vi "Dashboard Main.vi"() -> ()   [LabVIEW 2014]
uses:
  Program Files (x86)/National Instruments/LabVIEW 2014/examples/FRC/roboRIO/Vision/2015 Vision Example/Vision Support Code/Camera Types.ctl
  <vilib>/event_ctls.llb/eventvkey.ctl
  <vilib>/Rock Robotics/WPI/Dashboard/WPI_DashboardLogging Global.vi
  <vilib>/Rock Robotics/Network Tables/SD Write Number.vi
  <vilib>/Rock Robotics/Network Tables/SD Write Boolean.vi
  <vilib>/Utility/config.llb/Write Key (String).vi
  <vilib>/Utility/config.llb/Write Key (I32).vi
  <vilib>/Utility/config.llb/NI_LVConfig.lvlib
  <vilib>/vision/NI_Vision_Development_Module.lvlib
panel:
  out "Camera Image 6":T1(plugin-control)
  out "Image Message":string="Timeout in Camera Communications"
  in  "TCP":refnum<k5>
  in  "Rec Mode":enum32{"Stop", "Record", "Playback"}(radio)
  in  "Vision":u16(ring)=3 items=["Camera Off", "USB Camera SW", "USB Camera HW", "IP Camera"]
  out "Camera IP":string
  in  "Dashboard Tab":T2(tab)
  in  "Camera Settings":T3={"Frame Rate"=30, "Compression"=30, "Size"=1} {"Frame Rate" scale=1.0..30.0; "Size" items=["640x480", "320x240", "160x120"]}
  out "MotorChart R":cluster{"Numeric":dbl, "Numeric":dbl}(graph)
  out "MotorChart L":T4(graph)
  out "MotorSliders R":cluster{"MotorSlide1":dbl, "MotorSlide2":dbl} {"MotorSlide2" scale=-1.0..1.0 scale format="%#_2e"; "MotorSlide1" scale=-1.0..1.0 scale format="%#_2e"}
  out "MotorSliders L":T5 {"MotorSlide4 2" scale=0.0..14.0 scale format="%#_2e"; "MotorSlide2" scale=-1.0..1.0 scale format="%#_2e"; "MotorSlide1" scale=-1.0..1.0 scale format="%#_2e"}
  out "Gyro":dbl(knob) scale=0.0..360.0
  out "JS1 Z":dbl(slide) scale=-1.0..1.0 scale format="%#_2e"
  out "JS1 Graph":cluster{"X":dbl, "Y":dbl}[](graph)
  out "JS1 Buttons":T6
  out "JS2 Z":dbl(slide) scale=-1.0..1.0 scale format="%#_2e"
  out "JS2 Graph":cluster{"X":dbl, "Y":dbl}[](graph)
  out "JS2 Buttons":T6
  out "Mode":T7(ring)=enum."Auto Disabled"
  in  "DB Camera Config":bool
  out "fps":dbl format="%#.1g"
  out "Mbps":dbl format="%#.1g"
  out "Mbps 2":bool
  in  "Tiempo de Espera":dbl
  in  "Repetir":bool
  in  "Autonomo":dbl
  out "Found Totes":T8(array[cluster]) {"Normalized Rect"."Numeric 5" format="%#_2g"; "Normalized Rect"."Numeric 3" format="%#_2g"; "Normalized Rect"."Numeric 2" format="%#_2g"; "Normalized Rect"."Numeric" format="%#_2g"}
  out "Sorted Scores":T9(array[cluster]) {"Carpet" format="%#_3g"; "S" format="%#_3g"; "Trapezoid %" format="%#_3g"; "L" format="%#_3g"; "Area to CH" format="%#_3g"; "X" format="%#_3g"; "Y" format="%#_3g"}
  out "Detected Totes":T8(array[cluster]) {"Normalized Rect"."Numeric 5" format="%#_2g"; "Normalized Rect"."Numeric 3" format="%#_2g"; "Normalized Rect"."Numeric 2" format="%#_2g"; "Normalized Rect"."Numeric" format="%#_2g"}
  out "Sorted Scores Extracted":T9(array[cluster]) {"Carpet" format="%#_3g"; "S" format="%#_3g"; "Trapezoid %" format="%#_3g"; "L" format="%#_3g"; "Area to CH" format="%#_3g"; "X" format="%#_3g"; "Y" format="%#_3g"}
  out "Detected Totes Extracted":T8(array[cluster]) {"Normalized Rect"."Numeric 5" format="%#_2g"; "Normalized Rect"."Numeric 3" format="%#_2g"; "Normalized Rect"."Numeric 2" format="%#_2g"; "Normalized Rect"."Numeric" format="%#_2g"}
  out "ms to process":u32
  in  "Tote Color":T10={"Hue"={23.67058792990901, 53.0}, "Sat"={88.0, 255.0}, "Val"={60.0, 159.85714285714286}} {"Hue" scale=0.0..255.0 scale format="%#_3g"}
  in  "Carpet Color":T11(tab)
  in  "Red":T10={"Hue"={231.0, 14.0}, "Sat"={83.0, 255.0}, "Val"={52.5, 255.0}} {"Hue" scale=0.0..255.0 scale format="%#_3g"}
  in  "Blue":T10={"Hue"={119.0, 181.0}, "Sat"={33.0, 255.0}, "Val"={48.571428571428584, 255.0}} {"Hue" scale=0.0..255.0 scale format="%#_3g"}
  in  "Annotate":bool=TRUE
  in  "Show Carpet Mask":bool=TRUE
  in  "Limit Tests?":bool=TRUE
  out "Particles":i32
  in  "Score Threshold":dbl=75.0
  in  "Aspect Fudge Factor":dbl=1.0
  in  "Camera Type":T12=enum."MS HD3000 square"
  out "Particles 2":i32
  in  "DB/String 9":string
  in  "DB/String 8":string
  in  "DB/String 7":string
  in  "DB/String 6":string
  in  "DB/String 5":string
  in  "DB/String 4":string
  in  "DB/String 3":string
  in  "DB/String 2":string
  in  "DB/String 1":string
  in  "DB/String 0":string
  in  "DB/Slider 0":dbl(slide) scale=0.0..5.0
  in  "DB/Slider 1":dbl(slide) scale=0.0..5.0
  in  "DB/Slider 2":dbl(slide) scale=0.0..5.0
  in  "DB/Slider 3":dbl(slide) scale=0.0..5.0
  out "DB/LED 3":bool
  out "DB/LED 2":bool
  out "DB/LED 1":bool
  out "DB/LED 0":bool
  in  "DB/Button 3":bool
  in  "DB/Button 2":bool
  in  "DB/Button 1":bool
  in  "DB/Button 0":bool caption="New Name"
  in  "Test Slider":dbl(slide) scale=0.0..100.0 scale format="%#_3g"
  in  "On/Off":bool caption="Solenoid"
  in  "Test Name":u16(ring) items=["Select the test to run...", "Example Test", "-------------------------------", "List of tests is built in robot code.", "Replace with your own automated tests."]
  in  "Test Tree":string(tree)
  in  "Motor":cluster{"Value":dbl, "Enable":bool} {"Value" scale=-1.0..1.0 scale format="%#_3g"}
  out "Progress":T13 {"Test Progress" scale=0.0..100.0}
  in  "Rev/Fwd":cluster{"Forward":bool, "Reverse":bool}
  in  "Test Ring":u16(ring) items=["Monochrome", "Color"]
  in  "Listbox":i32(listbox)
  out "Tree":string(tree)
  in  "Tab Control":T14(tab)
  out "Original Image":T1(plugin-control)
  out "Masked":T1(plugin-control)
  out "Original Extracted":T1(plugin-control)
  out "Extracted Masked":T1(plugin-control)
  out "Boolean":bool
  # "Left"
  # "Front"
  # "Right"
  # "Battery"
  # "Density Profile"
  # "Aspect Ratio"
  # "Density Profile"
  # "Aspect Ratio"
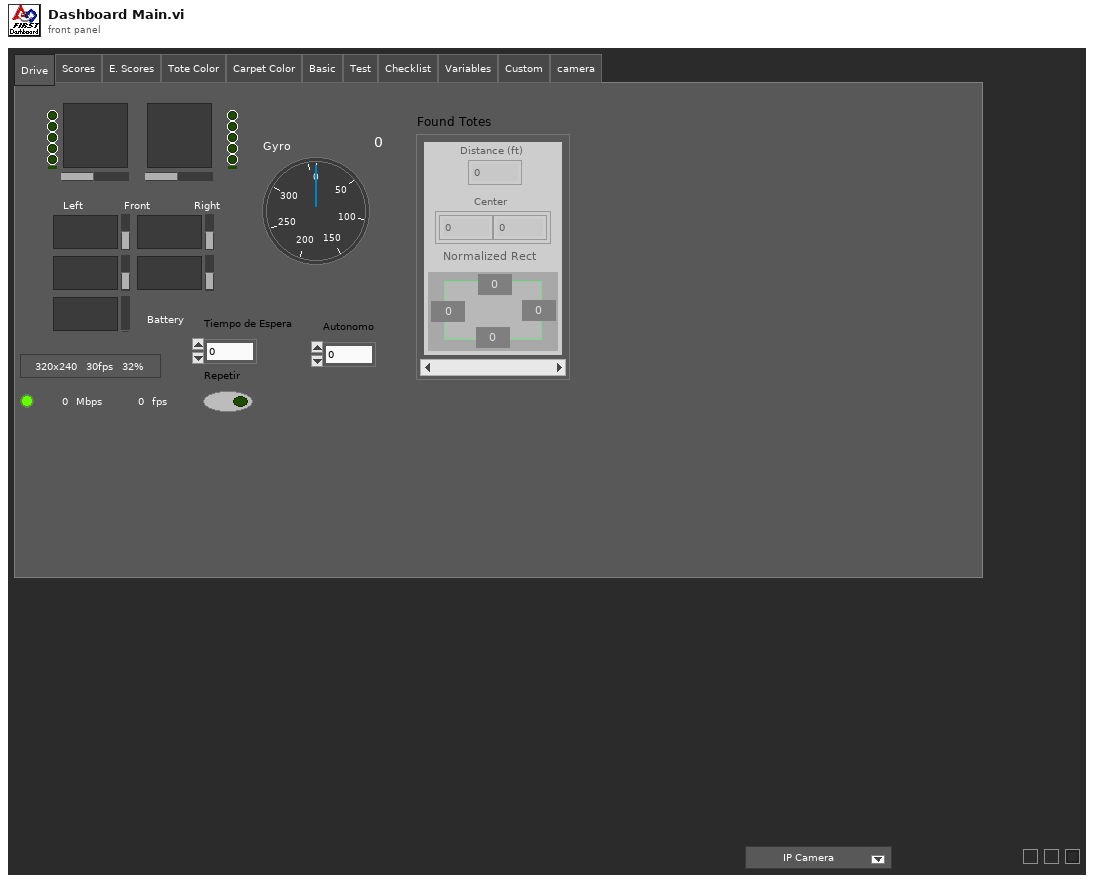
[diagram p1: front panel]
types:
  T1 = typedef "IMAQ Image.ctl" = refnum<image>
  T2 = enum32{"Drive", "Scores", "E. Scores", "Tote Color", "Carpet Color", "Basic", "Test", "Checklist", "Variables", "Custom", "camera"}
  T3 = cluster{"Frame Rate":i32, "Compression":i32, "Size":u16}
  T4 = cluster{"Numeric":dbl, "Numeric":dbl, "Battery V":dbl}
  T5 = cluster{"MotorSlide1":dbl, "MotorSlide2":dbl, "MotorSlide4 2":dbl}
  T6 = cluster{bool, bool, bool, bool, bool, bool, bool, bool, bool, bool, bool, bool}
  T7 = enum8{"Tele-Op Disabled", "Tele-Op Enabled", "Auto Disabled", "Auto Enabled", "Test Disabled", "Test Enabled", "Disconnected", "No Code", "E-Stop"}
  T8 = cluster{"Distance (ft)":dbl, "Center":cluster{dbl, dbl}, "Normalized Rect":cluster{"Numeric":dbl, "Numeric 2":dbl, "Numeric 3":dbl, "Numeric 5":dbl}}[]
  T9 = cluster{"Rectangle":cluster{"Numeric":dbl, "Numeric 2":dbl, "Numeric 3":dbl, "Numeric 5":dbl}, "Trapezoid %":dbl, "L":dbl, "S":dbl, "Area to CH":dbl, "X":dbl, "Y":dbl, "Carpet":dbl}[]
  T10 = cluster{"Hue":cluster{dbl, dbl}, "Sat":cluster{dbl, dbl}, "Val":cluster{dbl, dbl}}
  T11 = enum32{"Red Carpet Color", "Blue Carpet Color", "None"}
  T12 = typedef "Camera Types.ctl" = enum16{"206", "1011", "1013", "MS HD3000 square", "MS HD3000 640x480"}
  T13 = cluster{"Test Progress":u8, "Test Progress Text":string}
  T14 = enum32{"Original", "Masked", "Original Extracted", "Extracted Masked", "Rectangle"}
  T15 = typedef "Image Type" = u32
  T16 = typedef "Particle Parameters" = i32
  T17 = enum32{"Drive", "Basic", "Custom", "Test", "Checklist", "Variables"}
  T18 = cluster{"Camera Image 6":refnum<vi>, "Dashboard Tab":refnum<vi>, "Boolean":refnum<vi>, "Vision":refnum<vi>, "Rec Mode":refnum<vi>, "Test Slider":refnum<vi>, "On/Off ":refnum<vi>, "Test Ring":refnum<vi>, "Rev/Fwd":refnum<vi>, "Test Name":refnum<vi>, "Motor":refnum<vi>, "Progress":refnum<vi>, "CheckList":refnum<vi>, "Tree":refnum<vi>, "Test Tree":refnum<vi>}
  T19 = cluster{"Error Strings":string, "Disable Counts":cluster{u16, u16}, "Rail Faults":cluster{u16, u16, u16}, "Robot IP":string, "DB Mode":u8, "Event Info":cluster{"Name":string, "Type":u8, "Number":u16, "Replay":u8}, "Camera Addr":string}
  T20 = cluster{"Storage":cluster{"Disk Free":u64, "RAM Block":u32, "RAM free":u32}, "CPU Utilization":cluster{"CPU % ISR":sgl, "CPU % Time Crit":sgl, "CPU % Timed Str":sgl, "CPU % High":sgl, "CPU % Above":sgl, "CPU % Normal":sgl, "CPU % Low":sgl}, "CAN":cluster{"% Bus Utilization":sgl, "Bus Off Cnt":u32, "TX_FIFO Full Cnt":u32, "Receive Error Cnt":u8, "Transmit Error Cnt":u8}, "HID":cluster{"HID Outputs":u32, "Rumble Low":u16, "Rumble High":u16}[]}
  T21 = cluster{"Status bits":cluster{"Test Mode":bool, "Autonomous":bool, "Enabled":bool, "Code Start":bool, "Brownout":bool, "Reserved 2":bool, "Reserved 3":bool, "E-Stop":bool}, "Code Trace":cluster{"Disabled":bool, "TeleOp":bool, "Auto":bool, "Test":bool}, "Controller Type":enum16{"unknown", "cRIO", "roboRio"}, "Code?":enum16{"unknown", "noCode", "code"}, "Battery V":dbl}
  T22 = cluster{"Control Bits":cluster{"TestMode":bool, "Autonomous":bool, "Enabled":bool, "FMS Present":bool, bool, bool, bool, "E-Stop":bool}, "Team Station ":u8, "Countdown":sgl, "Joystick Values":cluster{"Axes":dbl[], "Buttons":bool[], "POVs":i16[]}[]}
  T23 = cluster{"Axes":dbl[], "Buttons":bool[], "POVs":i16[]}[]
  T24 = cluster{"Axes":dbl[], "Buttons":bool[], "POVs":i16[]}
  T25 = cluster{"Buttons[0]":bool, "Buttons[1]":bool, "Buttons[2]":bool, "Buttons[3]":bool, "Buttons[4]":bool, "Buttons[5]":bool, "Buttons[6]":bool, "Buttons[7]":bool, "Buttons[8]":bool, "Buttons[9]":bool, "Buttons[10]":bool, "Buttons[11]":bool}
  T26 = typedef "NI_LVConfig.lvlib/Config Data RefNum.ctl" = refnum<k1>
  T27 = cluster{"Operation":enum16{"Update", "Clear"}, "Color Box":u32}[]
  T28 = typedef "eventvkey.ctl" = enum16{"ASCII", "Enter", "Return", "Shift", "Ctrl", "Alt", "Cmd", "Opt", "Caps", "NumLock", "Clear", "Break", "Up", "Down", "Left", "Right", "Insert", "Delete", "Home", "End", "PageUp", "PageDown", "Escape", "Help", "Pause", "ScrollLock", "F1", "F2", "F3", "F4", "F5", "F6", "F7", "F8", "F9", "F10", "F11", "F12", "F13", "F14", "F15", "F16", "F17", "F18", "F19", "F20", "F21", "F22", "F23", "F24", "Play", "VolumeUp", "VolumeDown", "Mute", "Two Byte Char"}
  T29 = cluster{"Image Size":bool, "Image Type":bool, "Pixel Value":bool, "ROI Information":bool, "Zoom Factor":bool}
  T30 = enum8{"Enabled", "Disabled", "Disabled and Grayed Out"}
  T31 = cluster{"Operation":enum16{"Update", "Clear"}, "Color Box":u32}
  T32 = cluster{"Bounding box":cluster{"left":dbl, "top":dbl, "right":dbl, "bottom":dbl}, "Trapezoid":dbl, "Long Aspect":dbl, "Short Aspect":dbl, "Area to CH":dbl, "X Mask":dbl, "Y Mask":dbl, "Carpet":dbl}[]
  T33 = cluster{"Red":cluster{"Hue":cluster{dbl, dbl}, "Sat":cluster{dbl, dbl}, "Val":cluster{dbl, dbl}}, "Blue":cluster{"Hue":cluster{dbl, dbl}, "Sat":cluster{dbl, dbl}, "Val":cluster{dbl, dbl}}}
  T34 = cluster{cluster{"[0]":dbl, "[1]":dbl, "[2]":dbl, "[3]":dbl}, "Score":dbl, "Long Edge Score":dbl, "Short Edge Score":dbl, dbl, "X Score":dbl, "Y Score":dbl, "Carpet":dbl}[]
  T35 = cluster{"Found Totes[0]":cluster{"Distance (ft)":dbl, "Center":cluster{dbl, dbl}, "Normalized Rect":cluster{"Numeric":dbl, "Numeric 2":dbl, "Numeric 3":dbl, "Numeric 5":dbl}}, "Found Totes[1]":cluster{"Distance (ft)":dbl, "Center":cluster{dbl, dbl}, "Normalized Rect":cluster{"Numeric":dbl, "Numeric 2":dbl, "Numeric 3":dbl, "Numeric 5":dbl}}, "Found Totes[2]":cluster{"Distance (ft)":dbl, "Center":cluster{dbl, dbl}, "Normalized Rect":cluster{"Numeric":dbl, "Numeric 2":dbl, "Numeric 3":dbl, "Numeric 5":dbl}}, "Found Totes[3]":cluster{"Distance (ft)":dbl, "Center":cluster{dbl, dbl}, "Normalized Rect":cluster{"Numeric":dbl, "Numeric 2":dbl, "Numeric 3":dbl, "Numeric 5":dbl}}, "Found Totes[4]":cluster{"Distance (ft)":dbl, "Center":cluster{dbl, dbl}, "Normalized Rect":cluster{"Numeric":dbl, "Numeric 2":dbl, "Numeric 3":dbl, "Numeric 5":dbl}}, "Found Totes[5]":cluster{"Distance (ft)":dbl, "Center":cluster{dbl, dbl}, "Normalized Rect":cluster{"Numeric":dbl, "Numeric 2":dbl, "Numeric 3":dbl, "Numeric 5":dbl}}, "Found Totes[6]":cluster{"Distance (ft)":dbl, "Center":cluster{dbl, dbl}, "Normalized Rect":cluster{"Numeric":dbl, "Numeric 2":dbl, "Numeric 3":dbl, "Numeric 5":dbl}}, "Found Totes[7]":cluster{"Distance (ft)":dbl, "Center":cluster{dbl, dbl}, "Normalized Rect":cluster{"Numeric":dbl, "Numeric 2":dbl, "Numeric 3":dbl, "Numeric 5":dbl}}, "Found Totes[8]":cluster{"Distance (ft)":dbl, "Center":cluster{dbl, dbl}, "Normalized Rect":cluster{"Numeric":dbl, "Numeric 2":dbl, "Numeric 3":dbl, "Numeric 5":dbl}}}
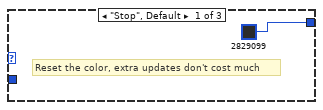
[diagram p3: hidden frame]
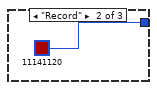
[diagram p4: hidden frame]
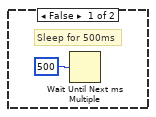
[diagram p6: hidden frame]
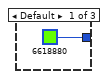
[diagram p7: hidden frame]
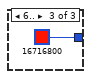
[diagram p8: hidden frame]
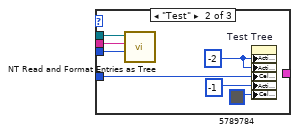
[diagram p10: hidden frame]
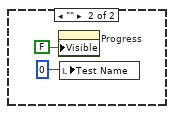
[diagram p11: hidden frame]
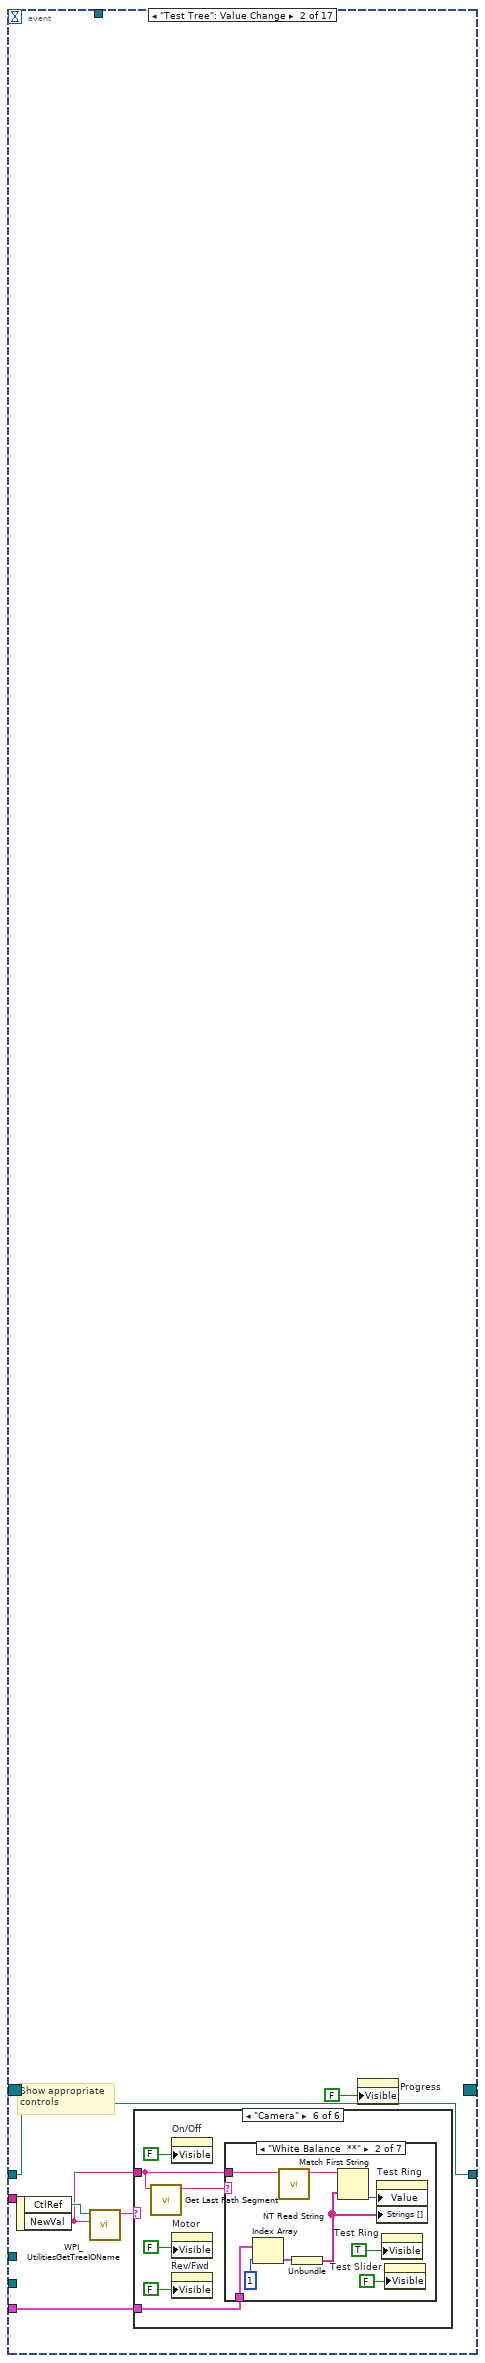
[diagram p12: hidden frame]
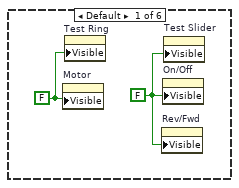
[diagram p13: hidden frame]
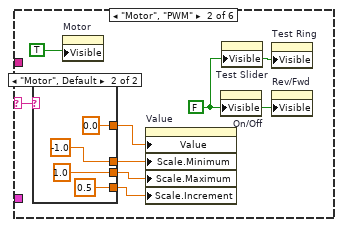
[diagram p14: hidden frame]
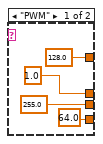
[diagram p15: hidden frame]
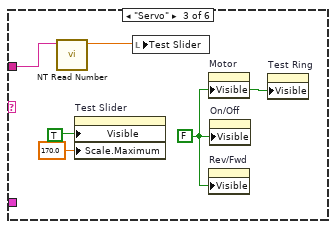
[diagram p16: hidden frame]
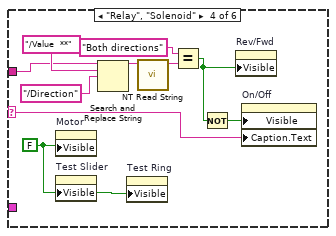
[diagram p17: hidden frame]
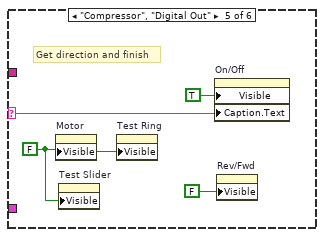
[diagram p18: hidden frame]
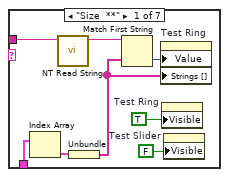
[diagram p19: hidden frame]
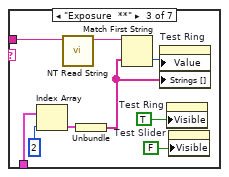
[diagram p20: hidden frame]
diagram:
  w5 = T15 0 items=["Grayscale (U8)", "Grayscale (I16)", "Grayscale (SGL)", "Complex (CSG)", "RGB (U32)", "HSL (U32)", "RGB (U64)"] ("Image Type")
  w7 = T15 4 items=["Grayscale (U8)", "Grayscale (I16)", "Grayscale (SGL)", "Complex (CSG)", "RGB (U32)", "HSL (U32)", "RGB (U64)", "Grayscale (U16)"] ("Image Type")
  w12 = T16[] [48, 35, 38, 4, 5, 6, 7, 0, 1, 2, 3] items=["Center of Mass X", "Center of Mass Y", "First Pixel X", "First Pixel Y", "Bounding Rect Left", "Bounding Rect Top", "Bounding Rect Right", "Bounding Rect Bottom", "Max Feret Diameter Start X", "Max Feret Diameter Start Y", "Max Feret Diameter End X", "Max Feret Diameter End Y", "Max Horiz. Segment Length Left", "Max Horiz. Segment Length Right", "Max Horiz. Segment Length Row", "-", "Bounding Rect Width", "Bounding Rect Height", "Bounding Rect Diagonal", "Perimeter", "Convex Hull Perimeter", "Holes' Perimeter", "Max Feret Diameter", "Equivalent Ellipse Major Axis", "Equivalent Ellipse Minor Axis", "Equivalent Ellipse Minor Axis (Feret)", "Equivalent Rect Long Side", "Equivalent Rect Short Side", "Equivalent Rect Diagonal", "Equivalent Rect Short Side (Feret)", "Average Horiz. Segment Length", "Average Vert. Segment Length", "Hydraulic Radius", "Waddel Disk Diameter", "-", "Area", "Holes' Area", "Particle & Holes' Area", "Convex Hull Area", "Image Area", "-", "Number of Holes", "Number of Horiz. Segments", "Number of Vert. Segments", "-", "Orientation", "Max Feret Diameter Orientation", "-", "% Area/Image Area", "% Area/(Particle & Holes' Area)", "Ratio of Equivalent Ellipse Axes", "Ratio of Equivalent Rect Sides", "-", "Elongation Factor", "Compactness Factor", "Heywood Circularity Factor", "Type Factor", "-", "Sum X", "Sum Y", "Sum XX", "Sum XY", "Sum YY", "Sum XXX", "Sum XXY", "Sum XYY", "Sum YYY", "-", "Moment of Inertia XX", "Moment of Inertia XY", "Moment of Inertia YY", "Moment of Inertia XXX", "Moment of Inertia XXY", "Moment of Inertia XYY", "Moment of Inertia YYY", "Norm. Moment of Inertia XX", "Norm. Moment of Inertia XY", "Norm. Moment of Inertia YY", "Norm. Moment of Inertia XXX", "Norm. Moment of Inertia XXY", "Norm. Moment of Inertia XYY", "Norm. Moment of Inertia YYY", "Hu Moment 1", "Hu Moment 2", "Hu Moment 3", "Hu Moment 4", "Hu Moment 5", "Hu Moment 6", "Hu Moment 7"]  # Requested Measurements
  w15 = T15 0 items=["Grayscale (U8)", "Grayscale (I16)", "Grayscale (SGL)", "Complex (CSG)", "RGB (U32)", "HSL (U32)", "RGB (U64)"] ("Image Type")
  w39 = 491  # min tab size
  w38 = 1.333  # min tab size
  w46 = enum32{"Stop", "Record", "Playback"}."Stop" ("Rec Mode")
  w22 = FALSE ("Visible")
  (unwired) "This VI has seven parallel loops for different tasks and a bit of initialization code that runs just once.\n\nTypical dashboard extensions only need to edit the panel. Adding new indicators or controls simply involves placing them on the panel in the Operations tab and naming them the same as the SmartDashboard variable on the robot\n\nIf the display needs to process the data before display, loop one is an example of doing that for the joysticks and motors.\n\nIf you want customize the video display or perform processing on it, loop two is where that takes place.\n\nOther loops should not need to be modified. They are pretty standard, and document the task they perform."  # Documentation
  w65 = T15 4 items=["Grayscale (U8)", "Grayscale (I16)", "Grayscale (SGL)", "Complex (CSG)", "RGB (U32)", "HSL (U32)", "RGB (U64)"] ("Image Type")
  # "Loop 7. Wait for DS connections"
  # "Basic debug and auto controls: Their data names are fixed, but\nthe displayed name, called a caption, can be changed directly or in\nrobot code such as shown in Begin."
  # "Controls for Test Mode, Camera Settings, etc."
  # "Additional UI Initialization"
  # "Loop 6. Animation for background of window during playback and record"
  # "Fires each time robot IP\nchanges, simulator does this"
  # "Fires each time window\ndocking changes."
  # "Collects all controls and indicators\nin the Basic and Custom tab.\nIf you need to bind additional controls,\nadd their references. You can extend the\nenum constant or use an integer."
  # "The remaining code below this line typically doesn't need to be modified."
  # "Loop 4. Process UI events related to test mode, checklist, and camera settings"
  # "Terminals of controls and indicators that are bound to the smart dashboard by name.\nYou can place the terminals anywhere you like and even read data from them.\nYou bind controls by adding the control reference to the array on the left. The subVI will\ndo this for the contents of a tab, and you can do it for individual items too, as shown with\nthe LED. To create get the reference, right-click and Create>>Reference."
  # "Loop 3. Wait until the robot response provides\n the Robot IP address.\nOnce known, bind controls and\nvariables with the same names."
  # "Loop 5. Adjusts placement onscreen, hides the titlebar, etc."
  # "Loop 1. Receive various data streams from Driver Station, update joystick, motors, and more complex displays that don't easily bind to variables."
  # "Loop 2. Receive camera images from Robot, update Mbps, fps, and do any processing or display"
  n1 = control-ref of="Camera Image 6"() -> (w10:refnum<vi>)
  n2 = control-ref of="Rec Mode"() -> (w28:refnum<vi>)
  n3 = control-ref of="Tree"() -> (w32:refnum<vi>)
  n4 = control-ref of="Test Tree"() -> (w31:refnum<vi>)
  n5 = control-ref of="Dashboard Tab"() -> (w41:refnum<vi>)
  n6 = control-ref of="Boolean"() -> (w36:refnum<vi>)
  n7 = control-ref of="On/Off"() -> (w26:refnum<vi>)
  n8 = control-ref of="Progress"() -> (w23:refnum<vi>)
  n9 = control-ref of="Rev/Fwd"() -> (w24:refnum<vi>)
  n10 = control-ref of="Motor"() -> (w29:refnum<vi>)
  n11 = control-ref of="Dashboard Tab"() -> (w44:refnum<vi>)
  n12 = control-ref of="Test Slider"() -> (w27:refnum<vi>)
  n13 = control-ref of="Vision"() -> (w40:refnum<vi>)
  n14 = control-ref of="Test Ring"() -> (w25:refnum<vi>)
  n15 = control-ref of="Test Name"() -> (w30:refnum<vi>)
  n16 = property class="VI" props=["Front Panel.Closeable"]() -> (reference out=w45:refnum<vi>)  [unwired: 2 in, 2 out]
  n17 = control-ref of="CheckList"() -> (w33:refnum<vi>)
  n18 = Bundle("min tab size"=w39, "min tab size"=w38) -> (w37:cluster{"min tab size":i32, "min tab size":dbl})  [unwired: 1 in]
  n19 = Obtain Notifier(name (unnamed)="Window Mode", notification data type=TRUE) -> (notifier out=w19:refnum<notifier>)  [unwired: 2 in, 2 out]
  n20 = call <vilib>:"Get Tab Control Refs.vi"("Page Index"=T17."Basic" ("Dashboard Tab"), "TabControl in"=w44) -> ("ControlsOnPage"=w20:refnum<vi>[])  [unwired: 9 in]
  n21 = call <vilib>:"Get Tab Control Refs.vi"("Page Index"=T17."Custom" ("Dashboard Tab"), "TabControl in"=w44) -> ("ControlsOnPage"=w43:refnum<vi>[])  [unwired: 9 in]
  n22 = Obtain Notifier(name (unnamed)="Robot IP Update", notification data type="IP Addr" ("name (unnamed)")) -> (notifier out=w21:refnum<notifier>)  [unwired: 2 in, 2 out]
  n23 = Bundle("Camera Image 6"=w10, "Dashboard Tab"=w41, "Boolean"=w36, "Vision"=w40, "Rec Mode"=w28, "Test Slider"=w27, "On/Off"=w26, "Test Ring"=w25, "Rev/Fwd"=w24, "Test Name"=w30, "Motor"=w29, "Progress"=w23, "CheckList"=w33, "Tree"=w32, "Test Tree"=w31) -> (w11:T18)  [unwired: 1 in]
  n24 = while {
    tunnel: [w77] -> _
    tunnel: w21 -> [w71]
    tunnel: w20 -> [w70]
    tunnel: w19 -> [w66]
    i -> [w77]
    stop <- FALSE stop-if-true
    n25 = local read "Vision"() -> (w68:u16)
    n26 = call <vilib>:"WPI_DashboardUpdateNames.vi"("Controls on Tab"=w70) -> ()  [unwired: 11 in]
    n27 = call <vilib>:"WPI_DashboardRetrieveStatusInfo.vi"("Vision"=w68, "Binding Refnum"=w71, "Window Mode Notifier"=w66, "TCP Cnx"="TCP") -> ("Power and Errors"=w72:T19, "Robot Metrics"=w75:T20, "Status Info"=w76:T21, "Control Info"=w73:T22, "Robot Mode"=w69:T7, "Process?"=w74:bool)  [unwired: 2 in]
    "Mode" <- w69
    n28 = case shown="True" w74 {
      tunnel: w76 -> [_ w103]
      tunnel: w75 -> [_ w102]
      tunnel: w73 -> [_ w101]
      tunnel: w72 -> [_ w100]
      tunnel: w69 -> [_ _]
      frame False {
      }
      frame True {
        # "swap motors to match\ncharts and include battery"
        n29 = Unbundle By Name(w101) -> ("Joystick Values"=w88:T23)  [unwired: 1 out]
        n30 = Unbundle By Name(w100) -> ("Camera Addr"=→"Camera IP":string)  [unwired: 1 out]
        n31 = Unbundle By Name(w102) -> ()  [unwired: 1 out]
        n32 = Unbundle By Name(w103) -> ("Battery V"=w89:dbl)  [unwired: 1 out]
        n33 = call <vilib>:"SD Read Numeric Array.vi"("Name"="RobotDrive Motors") -> ("Numeric Array"=w91:dbl[])  [unwired: 8 in, 2 out]
        n34 = Index Array(array=w91, index #1=1, index #4=0) -> (element #1=w95:dbl, element #2=w96:dbl, element #3=w94:dbl, element #4=w99:dbl)  [unwired: 2 in]
        n35 = Index Array(array=w88) -> (element #1=w87:T24, element #2=w82:T24)  [unwired: 2 in]
        n36 = call "Prepare Joystick Data for Displays.vi"("Joystick Values"=w82) -> ("Buttons"=→"JS2 Buttons":T25, "Z Axis"=→"JS2 Z":dbl, "Cartesian Data"=→"JS2 Graph":cluster{"X axis":dbl, "X axis":dbl}[])  [unwired: 8 in]
        n37 = call "Prepare Joystick Data for Displays.vi"("Joystick Values"=w87) -> ("Buttons"=→"JS1 Buttons":T25, "Z Axis"=→"JS1 Z":dbl, "Cartesian Data"=→"JS1 Graph":cluster{"X axis":dbl, "X axis":dbl}[])  [unwired: 8 in]
        n38 = Bundle("Numeric"=w94, "Numeric"=w95) -> (→"MotorChart R" →"MotorSliders R":cluster{"Numeric":dbl, "Numeric":dbl})  [unwired: 1 in]
        n39 = Bundle("Numeric"=w96, "Numeric"=w99, "Battery V"=w89) -> (→"MotorChart L" →"MotorSliders L":T4)  [unwired: 1 in]
      }
    }
  }
  n40 = Build Array (concatenate)(w20, w43) -> (w42:refnum<vi>[])
  n41 = call "Adjust Dashboard Window.vi"("Sizing Refnums"=w11, "Size Constraints"=w37, "VI"=w45, "Notifier in"=w19) -> ()  [unwired: 8 in]
  n42 = register-events(refnum<vi> refnum) -> (reference out=w50:refnum<event-registration>, error out=w49:errorcluster)  [unwired: 2 in]
  n43 = property class="VI"() -> ("Panel"=w53:refnum<vi>)  [unwired: 2 in, 2 out]
  n44 = while {
    tunnel: w42 -> [w115]
    tunnel: w21 -> [w113]
    tunnel: [w111] -> _
    tunnel: u32 1000 ("milliseconds to wait") -> [w110]
    i -> [w111]
    stop <- FALSE stop-if-true
    n45 = local read "Rec Mode"() -> (w106:enum32{"Stop", "Record", "Playback"})
    n46 = Wait on Notification(notifier=w113, timeout in ms (-1)=w110) -> (notification=w112:string, timed out?=w108:bool)  [unwired: 2 in, 2 out]
    n47 = Equal?(x=w106, y=u16 2 ("Rec Mode")) -> (x = y?=w107:bool)
    n48 = Compound Arithmetic op=OR(invert w108, w107) -> (w109:bool)
    n49 = case shown="True" w109 {
      tunnel: w115 -> [_ w118]
      tunnel: w112 -> [_ w117]
      tunnel: "Dashboard" -> [_ w116]
      frame False {
      }
      frame True {
        n50 = call <vilib>:"Bind Controls to SmartDashboard.vi"("Client Name"=w116, "Bound Control Refs"=w118, "Server IP Address"=w117) -> ()  [unwired: 9 in]
      }
    }
  }
  n51 = vi-ref "Playback Controls.vi"() -> (w51:refnum<vi>)
  n52 = call "Initialize Camera and CheckList.vi"("ListBox in"=w33) -> ("Cluster"=w57:cluster{"value":i32, "value":i32, "index":i32}, "Array"=w58:cluster{string[]}[], "File Refnum"=w56:T26)  [unwired: 8 in]
  n53 = property class="Pnl"(reference=w53) -> ("Panes[]"=w54:refnum<vi>[])  [unwired: 1 in, 2 out]
  n54 = property on="Camera Settings" class="Clust (strict)"("Val(Sgnl)"=w57) -> ()  [unwired: 2 in, 2 out]
  n55 = Index Array(array=w54) -> (element=w52:refnum<vi>)  [unwired: 1 in]
  n56 = control-ref of="Test Tree"() -> (w55:refnum<vi>)
  n57 = while {
    tunnel: w58 -> [w126]
    shift-right: [w125] -> _
    shift-left: w56 -> [w124]
    tunnel: [w123] -> _
    tunnel: w55 -> [w122]
    tunnel: w51 -> [w121]
    tunnel: w50 -> [w120]
    tunnel: w49 -> [_]
    tunnel: w45 -> [w119]
    i -> [w123]
    stop <- FALSE stop-if-true
    n58 = event shown="[0] Timeout" {
      selector: w120 -> [_ _ _ _ _ _ _ _ _ _ _ _ _ _ _ _ _]
      dyn-events: [_ _ _ _ _ _ _ _ _ _ _ _ _ w362 _ _ _] -> _
      timeout: u32 60 ("milliseconds to wait") -> [_ _ _ _ _ _ _ _ _ _ _ _ _ _ _ _ _]
      tunnel: w122 -> [w138 _ _ _ _ _ _ _ _ _ _ _ _ _ _ _ _]
      tunnel: "Test Tree" -> [_ _ _ _ _ _ _ _ w333 w341 w343 w347 w355 _ _ _ _]
      tunnel: w126 -> [_ w160 _ _ _ _ w297 w327 _ _ _ _ _ _ _ _ _]
      tunnel: [w134 w159 w258 w263 w271 w283 w296 w320 w332 w339 w342 w346 w354 w364 w378 w379 w389] -> w125
      tunnel: w124 -> [w134 w159 w258 w263 w271 w283 w295 w320 w332 w339 w342 w346 w354 w364 w378 w379 w389]
      tunnel: w121 -> [_ _ _ _ _ _ _ _ _ _ _ _ _ w365 _ w382 _]
      tunnel: w119 -> [_ _ _ _ _ _ _ _ _ _ _ _ _ w360 _ _ _]
      event Timeout {
        n59 = event-data() -> ()  [unwired: 1 in, 1 out]
        n60 = local read "Mode"() -> (w137:T7)
        n61 = Index Array(array=T27 [{"Operation"=enum."Clear", "Color Box"=14013909}, {"Operation"=enum."Clear", "Color Box"=14013909}, {"Operation"=enum."Clear", "Color Box"=14013909}, {"Operation"=enum."Clear", "Color Box"=14013909}, {"Operation"=enum."Update", "Color Box"=14013909}, {"Operation"=enum."Update", "Color Box"=16777215}, {"Operation"=enum."Clear", "Color Box"=14013909}, {"Operation"=enum."Clear", "Color Box"=14013909}, {"Operation"=enum."Clear", "Color Box"=14013909}], index=w137) -> (element=w132:T31)
        n62 = Unbundle(w132) -> ("Operation"=w131:enum16{"Update", "Clear"}, "Color Box"=w130:u32)
        n63 = call <vilib>:"NT Read String.vi"("Name"="TestMode/TestName") -> ("String"=w141:string)  [unwired: 9 in, 1 out]
        n64 = case shown="\"Variables\"" "Dashboard Tab" {
          tunnel: w138 -> [_ w149 _]
          tunnel: "/TestMode/Automatic/" ("Name Pattern") -> [_ w148 _]
          tunnel: w131 -> [_ w147 _]
          tunnel: [_ _ w151] -> _
          tunnel: w130 -> [_ w143 _]
          frame "Custom", Default {
          }
          frame "Test" {
            w146 = -2 ("Active Item:Row Number")
            n65 = call <vilib>:"NT Read and Format Entries as Tree.vi"("Operation"=w147, "Name Pattern"=w148, "Tree Refnum"=w149) -> ()  [unwired: 7 in, 2 out]
            n66 = property on="Test Tree" class="Tree (strict)"("Active Item Row Number"=w146, "ActiveColNum"=w146, "CellBG"=w143, "Active Item Row Number"=-1 ("Active Item:Row Number"), "CellBG"=u32 5789784 ("Color Box")) -> ()  [unwired: 2 in, 2 out]
          }
          frame "Variables" {
            n67 = control-ref of="Tree"() -> (w150:refnum<vi>)
            n68 = call <vilib>:"NT Read and Format Entries as Tree.vi"("Tree Refnum"=w150) -> ("Formatted Strings"=w151:cluster{"Name":string, "Value":string}[])  [unwired: 9 in, 1 out]
          }
        }
        n69 = case shown="Default" w141 {
          tunnel: "TestMode/TestProgress" ("Name") -> [w153 _]
          tunnel: "TestMode/TestProgressText" ("Name") -> [w152 _]
          frame Default {
            n70 = call <vilib>:"NT Read Number.vi"("Name"=w153) -> ("Numeric"=w154:dbl)  [unwired: 9 in, 1 out]
            n71 = call <vilib>:"NT Read String.vi"("Name"=w152) -> ("String"=w155:string)  [unwired: 9 in, 1 out]
            n72 = Bundle("Numeric"=w154, "String"=w155) -> (→"Progress":cluster{"Numeric":dbl, "String":string})  [unwired: 1 in]
          }
          frame "" {
            n73 = property on="Progress" class="Clust (strict)"("Visible"=FALSE) -> ()  [unwired: 2 in, 2 out]
            n74 = local write "Test Name"(u16 0) -> ()
          }
        }
      }
      event "Test Tree": Value Change {
        # "Show appropriate\ncontrols"
        n75 = event-data() -> ("CtlRef"=w163:refnum<vi>, "NewVal"=w161:string)  [unwired: 1 in]
        n76 = call <vilib>:"WPI_UtilitiesGetTreeIOName.vi"("NewVal"=w161, "TreeControl in"=w163) -> ("I/O Name"=w164:string)  [unwired: 9 in]
        n77 = case shown="\"Camera\"" w164 {
          selector: w164 -> [_ w171 _ w189 w198 _]
          tunnel: w161 -> [_ _ w186 w188 _ w205]
          tunnel: w160 -> [_ _ _ _ _ w204]
          frame Default {
            w166 = FALSE ("Visible")
            w165 = FALSE ("Visible")
            n78 = property on="Motor" class="Clust (strict)"("Visible"=w165) -> ()  [unwired: 2 in, 2 out]
            n79 = property on="Test Ring" class="Ring (strict)"("Visible"=w165) -> ()  [unwired: 2 in, 2 out]
            n80 = property on="Rev/Fwd" class="Clust (strict)"("Visible"=w166) -> ()  [unwired: 2 in, 2 out]
            n81 = property on="On/Off" class="Bool (strict)"("Visible"=w166) -> ()  [unwired: 2 in, 2 out]
            n82 = property on="Test Slider" class="Slide (strict)"("Visible"=w166) -> ()  [unwired: 2 in, 2 out]
          }
          frame "Motor", "PWM" {
            w172 = FALSE ("Visible")
            n83 = case shown="\"Motor\", Default" w171 {
              tunnel: [1.0 ("Value") -1.0 ("Value")] -> w170
              tunnel: [255.0 ("Value") 1.0 ("Value")] -> w169
              tunnel: [128.0 ("Value") 0.0 ("Value")] -> w168
              tunnel: [64.0 ("Value") 0.5 ("Value")] -> w167
              frame "PWM" {
              }
              frame "Motor", Default {
              }
            }
            n84 = property on="Motor" class="Clust (strict)"("Visible"=TRUE) -> ()  [unwired: 2 in, 2 out]
            n85 = property on="Value" class="Slide (strict)"("Value"=w168, "Scale.Minimum"=w170, "Scale.Maximum"=w169, "Scale.Increment"=w167) -> ()  [unwired: 2 in, 2 out]
            n86 = property on="On/Off" class="Bool (strict)"("Visible"=w172) -> ()  [unwired: 2 in, 2 out]
            n87 = property on="Test Slider" class="Slide (strict)"("Visible"=w172) -> ()  [unwired: 2 in, 2 out]
            n88 = property on="Test Ring" class="Ring (strict)"("Visible"=w172) -> ()  [unwired: 2 in, 2 out]
            n89 = property on="Rev/Fwd" class="Clust (strict)"("Visible"=w172) -> ()  [unwired: 2 in, 2 out]
          }
          frame "Servo" {
            w184 = FALSE ("Visible")
            n90 = call <vilib>:"NT Read Number.vi"("Name"=w186) -> ("Numeric"=w185:dbl)  [unwired: 9 in, 1 out]
            n91 = property on="Test Slider" class="Slide (strict)"("Visible"=TRUE, "Scale.Maximum"=170.0 ("Scale.Range:Maximum")) -> ()  [unwired: 2 in, 2 out]
            n92 = local write "Test Slider"(w185) -> ()
            n93 = property on="Motor" class="Clust (strict)"("Visible"=w184) -> ()  [unwired: 2 in, 2 out]
            n94 = property on="Rev/Fwd" class="Clust (strict)"("Visible"=w184) -> ()  [unwired: 2 in, 2 out]
            n95 = property on="On/Off" class="Bool (strict)"("Visible"=w184) -> ()  [unwired: 2 in, 2 out]
            n96 = property on="Test Ring" class="Ring (strict)"("Visible"=w184) -> ()  [unwired: 2 in, 2 out]
          }
          frame "Relay", "Solenoid" {
            w187 = FALSE ("Visible")
            n97 = property on="Motor" class="Clust (strict)"("Visible"=w187) -> ()  [unwired: 2 in, 2 out]
            n98 = property on="Test Slider" class="Slide (strict)"("Visible"=w187) -> ()  [unwired: 2 in, 2 out]
            n99 = Search and Replace String(input string=w188, search string="/Value  **", replace string="/Direction") -> (result string=w194:string)  [unwired: 5 in, 3 out]
            n100 = property on="Test Ring" class="Ring (strict)"("Visible"=w187) -> ()  [unwired: 2 in, 2 out]
            n101 = call <vilib>:"NT Read String.vi"("Name"=w194) -> ("String"=w192:string)  [unwired: 9 in, 1 out]
            n102 = Equal?(x="Both directions", y=w192) -> (x = y?=w190:bool)
            n103 = Not(x=w190) -> (.not. x?=w191:bool)
            n104 = property on="Rev/Fwd" class="Clust (strict)"("Visible"=w190) -> ()  [unwired: 2 in, 2 out]
            n105 = property on="On/Off" class="Bool (strict)"("Visible"=w191, "Caption.Text"=w189) -> ()  [unwired: 2 in, 2 out]
          }
          frame "Compressor", "Digital Out" {
            w197 = FALSE ("Visible")
            # "Get direction and finish"
            n106 = property on="Motor" class="Clust (strict)"("Visible"=w197) -> ()  [unwired: 2 in, 2 out]
            n107 = property on="Test Slider" class="Slide (strict)"("Visible"=w197) -> ()  [unwired: 2 in, 2 out]
            n108 = property on="Test Ring" class="Ring (strict)"("Visible"=w197) -> ()  [unwired: 2 in, 2 out]
            n109 = property on="On/Off" class="Bool (strict)"("Visible"=TRUE, "Caption.Text"=w198) -> ()  [unwired: 2 in, 2 out]
            n110 = property on="Rev/Fwd" class="Clust (strict)"("Visible"=FALSE) -> ()  [unwired: 2 in, 2 out]
          }
          frame "Camera" {
            n111 = call <vilib>:"Get Last Path Segment.vi"("String in"=w205) -> ("String out"=w206:string)  [unwired: 10 in]
            n112 = property on="On/Off" class="Bool (strict)"("Visible"=FALSE) -> ()  [unwired: 2 in, 2 out]
            n113 = property on="Motor" class="Clust (strict)"("Visible"=FALSE) -> ()  [unwired: 2 in, 2 out]
            n114 = property on="Rev/Fwd" class="Clust (strict)"("Visible"=FALSE) -> ()  [unwired: 2 in, 2 out]
            n115 = case shown="\"White Balance  **\"" w206 {
              tunnel: w205 -> [w212 w221 w230 w239 w248 _ w254]
              tunnel: w204 -> [w210 w218 w227 w236 w245 _ _]
              frame "Size  **" {
                n116 = Index Array(array=w210) -> (element=w209:cluster{string[]})  [unwired: 1 in]
                n117 = call <vilib>:"NT Read String.vi"("Name"=w212) -> ("String"=w211:string)  [unwired: 9 in, 1 out]
                n118 = Unbundle(w209) -> (w207:string[])
                n119 = Match First String(2:w207, 3:w211) -> (0:w208:i32)  [unwired: 1 out]
                n120 = property on="Test Ring" class="Ring (strict)"("Value"=w208, "Strings []"=w207) -> ()  [unwired: 2 in, 2 out]
                n121 = property on="Test Ring" class="Ring (strict)"("Visible"=TRUE) -> ()  [unwired: 2 in, 2 out]
                n122 = property on="Test Slider" class="Slide (strict)"("Visible"=FALSE) -> ()  [unwired: 2 in, 2 out]
              }
              frame "White Balance  **" {
                n123 = Index Array(array=w218, index=1) -> (element=w219:cluster{string[]})
                n124 = call <vilib>:"NT Read String.vi"("Name"=w221) -> ("String"=w220:string)  [unwired: 9 in, 1 out]
                n125 = Unbundle(w219) -> (w216:string[])
                n126 = Match First String(2:w216, 3:w220) -> (0:w215:i32)  [unwired: 1 out]
                n127 = property on="Test Ring" class="Ring (strict)"("Value"=w215, "Strings []"=w216) -> ()  [unwired: 2 in, 2 out]
                n128 = property on="Test Ring" class="Ring (strict)"("Visible"=TRUE) -> ()  [unwired: 2 in, 2 out]
                n129 = property on="Test Slider" class="Slide (strict)"("Visible"=FALSE) -> ()  [unwired: 2 in, 2 out]
              }
              frame "Exposure  **" {
                n130 = Index Array(array=w227, index=2) -> (element=w228:cluster{string[]})
                n131 = call <vilib>:"NT Read String.vi"("Name"=w230) -> ("String"=w229:string)  [unwired: 9 in, 1 out]
                n132 = Unbundle(w228) -> (w224:string[])
                n133 = Match First String(2:w224, 3:w229) -> (0:w225:i32)  [unwired: 1 out]
                n134 = property on="Test Ring" class="Ring (strict)"("Value"=w225, "Strings []"=w224) -> ()  [unwired: 2 in, 2 out]
                n135 = property on="Test Ring" class="Ring (strict)"("Visible"=TRUE) -> ()  [unwired: 2 in, 2 out]
                n136 = property on="Test Slider" class="Slide (strict)"("Visible"=FALSE) -> ()  [unwired: 2 in, 2 out]
              }
              frame "Exposure Priority  **" {
                n137 = Index Array(array=w236, index=3) -> (element=w237:cluster{string[]})
                n138 = call <vilib>:"NT Read String.vi"("Name"=w239) -> ("String"=w238:string)  [unwired: 9 in, 1 out]
                n139 = Unbundle(w237) -> (w233:string[])
                n140 = Match First String(2:w233, 3:w238) -> (0:w234:i32)  [unwired: 1 out]
                n141 = property on="Test Ring" class="Ring (strict)"("Value"=w234, "Strings []"=w233) -> ()  [unwired: 2 in, 2 out]
                n142 = property on="Test Ring" class="Ring (strict)"("Visible"=TRUE) -> ()  [unwired: 2 in, 2 out]
                n143 = property on="Test Slider" class="Slide (strict)"("Visible"=FALSE) -> ()  [unwired: 2 in, 2 out]
              }
              frame "Color Enable  **" {
                n144 = Index Array(array=w245, index=4) -> (element=w246:cluster{string[]})
                n145 = call <vilib>:"NT Read String.vi"("Name"=w248) -> ("String"=w247:string)  [unwired: 9 in, 1 out]
                n146 = Unbundle(w246) -> (w242:string[])
                n147 = Match First String(2:w242, 3:w247) -> (0:w243:i32)  [unwired: 1 out]
                n148 = property on="Test Ring" class="Ring (strict)"("Value"=w243, "Strings []"=w242) -> ()  [unwired: 2 in, 2 out]
                n149 = property on="Test Ring" class="Ring (strict)"("Visible"=TRUE) -> ()  [unwired: 2 in, 2 out]
                n150 = property on="Test Slider" class="Slide (strict)"("Visible"=FALSE) -> ()  [unwired: 2 in, 2 out]
              }
              frame Default {
                n151 = property on="Test Ring" class="Ring (strict)"("Visible"=FALSE) -> ()  [unwired: 2 in, 2 out]
                n152 = property on="Test Slider" class="Slide (strict)"("Visible"=FALSE) -> ()  [unwired: 2 in, 2 out]
              }
              frame "Brightness  **", "Color Level  **", "Compression  **", "FPS  **", "Sharpness  **" {
                n153 = call <vilib>:"NT Read Number.vi"("Name"=w254) -> ("Numeric"=w253:dbl)  [unwired: 9 in, 1 out]
                n154 = local write "Test Slider"(w253) -> ()
                n155 = property on="Test Slider" class="Slide (strict)"("Visible"=TRUE, "Scale.Maximum"=100.0 ("Scale.Range:Maximum")) -> ()  [unwired: 2 in, 2 out]
                n156 = property on="Test Ring" class="Ring (strict)"("Visible"=FALSE) -> ()  [unwired: 2 in, 2 out]
              }
            }
          }
        }
        n157 = property on="Progress" class="Clust (strict)"("Visible"=FALSE) -> ()  [unwired: 2 in, 2 out]
      }
      event "Test Name": Mouse Enter {
        # "Populate the ring with the list of tests"
        n158 = event-data() -> ()  [unwired: 1 in, 1 out]
        n159 = call <vilib>:"NT Read String Array.vi"("Name"="TestMode/TestList") -> ("String Array"=w262:string[])  [unwired: 9 in, 1 out]
        n160 = Build Array (concatenate)("Select the test to run...", w262) -> (w261:string[])
        n161 = property on="Test Name" class="Ring (strict)"("Strings []"=w261) -> ()  [unwired: 2 in, 2 out]
      }
      event "Test Name": Value Change {
        w264 = FALSE ("Visible")
        # "Tell the robot the test name to run"
        n162 = event-data() -> ("NewVal"=w268:u16)  [unwired: 1 in]
        n163 = property on="Test Name" class="Ring (strict)"() -> ("Strings []"=w269:string[])  [unwired: 2 in, 2 out]
        n164 = local write "Progress"(T13 {"Test Progress"=0, "Test Progress Text"=""} ("Progress")) -> ()
        n165 = Index Array(array=w269, index=w268) -> (element=w267:string)
        n166 = call <vilib>:"NT Write String.vi"("String"=w267, "Name"="TestMode/TestName") -> ()  [unwired: 9 in, 1 out]
        n167 = property on="Progress" class="Clust (strict)"("Visible"=TRUE) -> ()  [unwired: 2 in, 2 out]
        n168 = property on="Motor" class="Clust (strict)"("Visible"=w264) -> ()  [unwired: 2 in, 2 out]
        n169 = property on="Test Slider" class="Slide (strict)"("Visible"=w264) -> ()  [unwired: 2 in, 2 out]
        n170 = property on="On/Off" class="Bool (strict)"("Visible"=w264) -> ()  [unwired: 2 in, 2 out]
        n171 = property on="Rev/Fwd" class="Clust (strict)"("Visible"=w264) -> ()  [unwired: 2 in, 2 out]
        n172 = property on="Test Ring" class="Ring (strict)"("Visible"=w264) -> ()  [unwired: 2 in, 2 out]
      }
      event "Listbox": Double Click {
        # "Shift clears all"
        # "Update symbols on the listbox"
        n173 = event-data() -> ("PlatMods.Shift"=w272:bool, "Row"=w274:i32)  [unwired: 1 in]
        n174 = case shown="True" w272 {
          tunnel: w274 -> [w278 _]
          tunnel: 1 -> [w277 _]
          frame False {
            n175 = property on="Listbox" class="LstBox (strict)"() -> ("Item Symbols"=w276:i32[])  [unwired: 2 in, 2 out]
            n176 = Replace Array Subset(array=w276, new element=w277, index=w278) -> (w275:i32[])
            n177 = property on="Listbox" class="LstBox (strict)"("Item Symbols"=w275) -> ()  [unwired: 2 in, 2 out]
          }
          frame True {
            w279 = 0 ("Top Row")
            n178 = property on="Listbox" class="LstBox (strict)"() -> ("Number of Rows"=w281:u32)  [unwired: 2 in, 2 out]
            n179 = Initialize Array(0, w281) -> (w280:i32[])
            n180 = property on="Listbox" class="LstBox (strict)"("Top Row"=w279, "Value"=w279, "Item Symbols"=w280) -> ()  [unwired: 2 in, 2 out]
          }
        }
      }
      event "Listbox": Key Down {
        # "Update symbols on the listbox\nLeft and right keys check and uncheck"
        n181 = event-data() -> ("VKey"=w285:T28)  [unwired: 1 in]
        n182 = case shown="\"Left\", \"Right\"" w285 {
          selector: w285 -> [w290 _]
          tunnel: eventvkey."Left" ("VKey") -> [w288 _]
          frame "Left", "Right" {
            n183 = Equal?(x=w288, y=w290) -> (x = y?=w289:bool)
            n184 = Select(t=0, s=w289, f=1) -> (s? t:f=w291:i32)
            n185 = property on="Listbox" class="LstBox (strict)"() -> ("Item Symbols"=w294:i32[])  [unwired: 2 in, 2 out]
            n186 = Replace Array Subset(array=w294, new element=w291, index="Listbox") -> (w293:i32[])
            n187 = property on="Listbox" class="LstBox (strict)"("Item Symbols"=w293) -> ()  [unwired: 2 in, 2 out]
          }
          frame Default {
          }
        }
      }
      event "DB Camera Config": Value Change {
        # "Show or hide the cluster of controls, store in ini file"
        n188 = event-data() -> ("NewVal"=w298:bool)  [unwired: 1 in]
        n189 = case shown="False" w298 {
          tunnel: w297 -> [w307 _]
          tunnel: [w300 w318] -> w296
          tunnel: w295 -> [w299 w318]
          frame False {
            w314 = "Camera"
            w317 = FALSE ("Visible")
            n190 = local read "Camera Settings"() -> (w306:T3)
            n191 = Index Array(array=w307) -> (element=w310:cluster{string[]})  [unwired: 1 in]
            n192 = Unbundle(w306) -> ("Frame Rate"=w305:i32, "Compression"=w304:i32, "Size"=w308:u16)
            n193 = Unbundle(w310) -> (w309:string[])
            n194 = Index Array(array=w309, index=w308) -> (element=w303:string)
            n195 = call-poly <vilib>:"Write Key.vi"("section"=w314, "value"=w303, "key"="Size", "refnum"=w299) -> ("refnum out"=w316:T26)  [unwired: 2 in, 5 out]
            n196 = call-poly <vilib>:"Write Key.vi"("section"=w314, "value"=w305, "key"="FrameRate", "refnum"=w316) -> ("refnum out"=w315:T26)  [unwired: 1 in, 6 out]
            n197 = property on="Camera Settings" class="Clust (strict)"("Visible"=w317) -> ()  [unwired: 2 in, 2 out]
            n198 = local write "DB Camera Config"(w317) -> ()
            n199 = call-poly <vilib>:"Write Key.vi"("section"=w314, "value"=w304, "key"="Compression", "refnum"=w315) -> ("refnum out"=w301:T26)  [unwired: 1 in, 6 out]
            n200 = call <vilib>:"Close Config Data.vi"("refnum"=w301) -> ("file path"=w302:path)  [unwired: 2 in, 8 out]
            n201 = call <vilib>:"Open Config Data.vi"("configuration file path"=w302) -> ("refnum"=w300:T26)  [unwired: 8 in, 2 out]
          }
          frame True {
            n202 = property on="Camera Settings" class="Clust (strict)"("Visible"=TRUE) -> ()  [unwired: 2 in, 2 out]
          }
        }
      }
      event "Camera Settings": Value Change {
        # "Update summary string when any elements of DB camera change"
        n203 = event-data() -> ("NewVal"=w331:T3)  [unwired: 1 in]
        n204 = Index Array(array=w327) -> (element=w326:cluster{string[]})  [unwired: 1 in]
        n205 = Unbundle(w331) -> ("Frame Rate"=w322:i32, "Compression"=w321:i32, "Size"=w324:u16)
        n206 = Unbundle(w326) -> (w325:string[])
        n207 = Index Array(array=w325, index=w324) -> (element=w323:string)
        n208 = Format Into String(format string="%s   %dfps   %d%%", w323, w322, w321) -> (resulting string=w328:string)  [unwired: 2 in, 1 out]
        n209 = Build Array(w328) -> (w329:string[])
        n210 = property on="DB Camera Config" class="Bool (strict)"("Strings [4]"=w329) -> ()  [unwired: 2 in, 2 out]
      }
      event "Motor.Enable": Value Change {
        # "When the test mode otor enable helper is set, update that\ntree row item's value"
        n211 = event-data() -> ("NewVal"=w337:bool)  [unwired: 1 in]
        n212 = Unbundle("Motor") -> ("Value"=w336:dbl)  [unwired: 1 out]
        n213 = Select(t=w336, s=w337, f=0.0) -> (s? t:f=w334:dbl)
        n214 = call <vilib>:"NT Write Number.vi"("Numeric"=w334, "Name"=w333) -> ()  [unwired: 9 in, 1 out]
      }
      event "Test Slider": Value Change {
        # "When the test mode slider helper is set, update that\ntree row item's value"
        n215 = event-data() -> ("NewVal"=w340:dbl)  [unwired: 1 in]
        n216 = call <vilib>:"NT Write Number.vi"("Numeric"=w340, "Name"=w341) -> ()  [unwired: 9 in, 1 out]
      }
      event "On/Off": Value Change {
        # "When the test mode on/off helper value is set, update that\ntree row item's value"
        n217 = event-data() -> ("NewVal"=w345:bool)  [unwired: 1 in]
        n218 = Boolean To (0,1)(Boolean=w345) -> (0, 1=w344:i16)
        n219 = call <vilib>:"NT Write Number.vi"("Numeric"=w344, "Name"=w343) -> ()  [unwired: 9 in, 1 out]
      }
      event "Rev/Fwd": Value Change {
        # "When the test mode helper value for relays is set, update that\ntree row item's value"
        n220 = event-data() -> ("NewVal.Forward"=w353:bool, "NewVal.Reverse"=w352:bool)  [unwired: 1 in]
        n221 = Boolean To (0,1)(Boolean=w353) -> (0, 1=w349:i16)
        n222 = Boolean To (0,1)(Boolean=w352) -> (0, 1=w351:i16)
        n223 = Negate(x=w351) -> (-x=w350:i16)
        n224 = Add(x=w349, y=w350) -> (x+y=w348:i16)
        n225 = call <vilib>:"NT Write Number.vi"("Numeric"=w348, "Name"=w347) -> ()  [unwired: 9 in, 1 out]
      }
      event "Test Ring": Value Change {
        # "When a test mode helper value is selected from the ring,\nset the tree item's variable to the string value"
        n226 = event-data() -> ("NewVal"=w357:u16)  [unwired: 1 in]
        n227 = property on="Test Ring" class="Ring (strict)"() -> ("Strings []"=w358:string[])  [unwired: 2 in, 2 out]
        n228 = Index Array(array=w358, index=w357) -> (element=w356:string)
        n229 = call <vilib>:"NT Write String.vi"("String"=w356, "Name"=w355) -> ()  [unwired: 9 in, 1 out]
      }
      event "Rec Mode": Value Change {
        # "Update globals for recording mode and path to read log from.\nClear when logging and let NetworkTables set path for vision to\nuse."
        n230 = event-data() -> ("NewVal"=w366:enum32{"Stop", "Record", "Playback"})  [unwired: 1 in]
        n231 = global write "WPI_DashboardLogging Global.vi" "Logging Filename"(path "") -> ()
        n232 = case shown="\"Playback\"" w366 {
          tunnel: w365 -> [_ w368 w376]
          tunnel: [_ _ w375] -> w362
          tunnel: [_ _ w374] -> _
          tunnel: w360 -> [_ _ w372]
          tunnel: cluster{i32, i32} {-250, 170} -> [_ _ w371]
          tunnel: [_ _ T29 {"Image Size"=TRUE, "Image Type"=TRUE, "Pixel Value"=TRUE, "ROI Information"=TRUE, "Zoom Factor"=FALSE} ("Image Information Shown:All Elements")] -> _
          tunnel: [_ _ TRUE ("Zoom Factor")] -> _
          frame Default {
          }
          frame "Stop", "Record" {
            # "Place Window too"
            n233 = invoke class="VI" method="FP.Close"(reference=w368) -> (reference out=w367:refnum<vi>)  [unwired: 2 in, 2 out]
            n234 = invoke class="VI" method="Abort VI"(reference=w367) -> ()  [unwired: 2 in, 3 out]
          }
          frame "Playback" {
            n235 = call "Open Playback Panel.vi"("Offset"=w371, "DB VI Ref"=w372, "Playback in"=w376) -> ("Playback out"=w373:refnum<vi>)  [unwired: 8 in]
            n236 = register-events(w373) -> (reference out=w375:refnum<event-registration>, error out=w374:errorcluster)  [unwired: 2 in]
          }
        }
        n237 = global write "WPI_DashboardLogging Global.vi" "Recording"(w366) -> ()
        n238 = call <vilib>:"WPI_DashboardNT Log FieldName Cache.vi"("Operation"=enum16{"Lookup/Add", "Index", "Clear"}."Clear") -> ()  [unwired: 8 in, 3 out]
      }
      event Panel Close {
        w377 = enum32{"Stop", "Record", "Playback"}."Stop" ("Rec Mode")
        # "Playback window has been closed, abort"
        n239 = event-data() -> ()  [unwired: 1 in, 4 out]
        n240 = local write "Rec Mode"(w377) -> ()
        n241 = global write "WPI_DashboardLogging Global.vi" "Recording"(w377) -> ()
      }
      event Panel Close {
        # "Abort playback window and ourself"
        n242 = event-data() -> ()  [unwired: 1 in, 4 out]
        n243 = invoke class="VI" method="FP.Close"(reference=w382) -> (reference out=w381:refnum<vi>)  [unwired: 2 in, 2 out]
        n244 = invoke class="VI" method="Abort VI"(reference=w381) -> (error out=w380:errorcluster)  [unwired: 2 in, 2 out]
        n245 = invoke class="VI" method="Abort VI"(error in=w380) -> ()  [unwired: 2 in, 3 out]
      }
      event "Vision": Value Change {
        # "Enable/Disable Compression slider.\nHW USB is hard-coded into the camera"
        n246 = event-data() -> ("NewVal"=w388:u16)  [unwired: 1 in]
        n247 = Equal?(x=w388, y=u32 2 ("milliseconds to wait")) -> (x = y?=w386:bool)
        n248 = Select(t=T30."Disabled and Grayed Out" ("Disabled"), s=w386, f=T30."Enabled" ("Disabled")) -> (s? t:f=w383:T30)
        n249 = property on="Compression" class="Slide (strict)"("DisabledEnum"=w383) -> ()  [unwired: 2 in, 2 out]
      }
    }
  }
  n250 = while {
    tunnel: w52 -> [w391]
    i -> [w394]
    stop <- FALSE stop-if-true
    n251 = Wait (ms)(milliseconds to wait=u32 100) -> ()  [unwired: 1 out]
    n252 = case shown="\"Playback\"" "Rec Mode" {
      tunnel: w394 -> [_ _ w409]
      tunnel: [u32 2829099 ("Base Color") u32 11141120 ("Target Color") w398] -> w390
      frame "Stop", Default {
        # "Reset the color, extra updates don't cost much"
      }
      frame "Record" {
      }
      frame "Playback" {
        # "Playback"
        n253 = Quotient & Remainder(x=w409, y=u32 50 ("milliseconds to wait")) -> (x-y*floor(x/y)=w405:u32)  [unwired: 1 out]
        n254 = Divide(x=w405, y=u32 50 ("milliseconds to wait")) -> (x/y=w402:dbl)
        n255 = Multiply(x=6.283185307179586, y=w402) -> (x*y=w407:dbl)
        n256 = Sine(x=w407) -> (sin(x)=w406:dbl)
        n257 = Absolute Value(x=w406) -> (abs(x)=w399:dbl)
        n258 = call "Interpolate RGB Color.vi"("Proportion"=w399, "Target Color"=u32 30976, "Base Color"=u32 2829099) -> ("Result Color"=w398:u32)  [unwired: 8 in]
      }
    }
    n259 = property class="Pane"(reference=w391, "PaneColor"=w390) -> ()  [unwired: 1 in, 2 out]
  }
  n260 = call "IMAQ Create"("Image Name"="Extracted Image", "Image Type"=w7) -> ("New Image"=w1:T1, "error out"=w2:errorcluster)  [unwired: 3 in]
  n261 = call "IMAQ Create"("Image Name"="Extracted Masked Image", "Image Type"=w5) -> ("New Image"=w4:T1, "error out"=w3:errorcluster)  [unwired: 2 in, 1 out]
  n262 = call "IMAQ Create"("Image Name"="Dashboard Image", "Image Type"=w65) -> ("New Image"=w16:T1, "error out"=w63:errorcluster)  [unwired: 2 in, 1 out]
  n263 = call "IMAQ Create"("Image Name"="Masked Image", "Image Type"=w15) -> ("New Image"=w13:T1, "error out"=w9:errorcluster)  [unwired: 2 in, 1 out]
  n264 = TCP Create Listener(10:u16 1741 ("timeout ms (25000)")) -> (3:w17:refnum<k5>)  [unwired: 4 in, 2 out]
  n265 = while {
    tunnel: w16 -> [w422]
    tunnel: w63 -> [_]
    tunnel: [w423] -> _
    tunnel: w13 -> [w414]
    tunnel: w12 -> [w413]
    tunnel: w9 -> [_]
    tunnel: w1 -> [w412]
    tunnel: w4 -> [w411]
    tunnel: w3 -> [_]
    tunnel: w2 -> [_]
    i -> [w423]
    stop <- FALSE stop-if-true
    n266 = local read "Rec Mode"() -> (w417:enum32{"Stop", "Record", "Playback"})
    n267 = call <vilib>:"WPI_CameraRead MJPG for Dashboard.vi"("Camera Settings"="Camera Settings", "Rec Mode"=w417, "Camera IP"="10.22.83.11", "Camera Mode"="Vision", "Refnum in"=w422) -> ("Active"=w421:bool, "Refnum out"=w410:T1, "FPS"=w420:dbl, "Bandwidth (Mbps)"=w419:dbl)  [unwired: 3 in]
    n268 = case shown="True" w421 {
      tunnel: w410 -> [_ w444]
      tunnel: w419 -> [_ w505]
      tunnel: w420 -> [_ w504]
      tunnel: w414 -> [_ w496]
      tunnel: w413 -> [_ w451]
      tunnel: w412 -> [_ w445]
      tunnel: w411 -> [_ w450]
      frame False {
        # "Sleep for 500ms"
        n269 = Wait Until Next ms Multiple(millisecond multiple=u32 500) -> ()  [unwired: 1 out]
      }
      frame True {
        w460 = 2.0  # Limit %
        w463 = 1.0  # Particles
        w458 = 4 ("Replace Value")
        w464 = u16 2 items=["RGB", "HSL", "HSV", "HSI"] ("Color Mode")
        w492 = 2.0  # Limit %
        w495 = 1.0  # Particles
        w486 = 4 ("Replace Value")
        w497 = u16 2 items=["RGB", "HSL", "HSV", "HSI"] ("Color Mode")
        # "Update Mbps LED"
        n270 = Tick Count (ms)() -> (millisecond timer value=w502:u32)
        n271 = case shown="4, 5" w505 {
          tunnel: [u32 6618880 ("Color Box") u32 16776722 ("Color Box") u32 16716800 ("Color Box")] -> w506
          frame Default {
          }
          frame 4, 5 {
          }
          frame 6.. {
          }
        }
        n272 = feedback #1() -> (w501:u32)  [unwired: 1 in]
        n273 = feedback-in #1(w502) -> ()
        n274 = call "IMAQ Clear Overlay"("Image"=w444) -> ("error out"=w509:errorcluster)  [unwired: 2 in, 8 out]
        n275 = Unbundle("Tote Color") -> ("Hue"=w498:cluster{dbl, dbl}, "Sat"=w499:cluster{dbl, dbl}, "Val"=w500:cluster{dbl, dbl})
        n276 = call-poly <vilib>:"SD Write Value.vi"("Boolean"="Repetir", "Name"="repetir") -> ()  [unwired: 8 in, 2 out]
        n277 = Unbundle By Name(w509) -> ("status"=w510:bool)
        n278 = Subtract(x=w502, y=w501) -> (x-y=→"ms to process":u32)
        n279 = Unbundle("Tote Color") -> ("Hue"=w465:cluster{dbl, dbl}, "Sat"=w466:cluster{dbl, dbl}, "Val"=w467:cluster{dbl, dbl})
        n280 = call "IMAQ Extract"("Y Step Size"=1, "Optional Rectangle"=i32[] [0, 366, 640, 480], "X Step Size"=1, "Image Dst"=w445, "Image Src"=w444) -> ("Image Dst Out"=w443:T1)  [unwired: 5 in, 1 out]
        n281 = call-poly <vilib>:"SD Write Value.vi"("Numeric"="Autonomo", "Name"="autonomo") -> ()  [unwired: 8 in, 2 out]
        n282 = property on="Image Message" class="Str"("Visible"=w510) -> ()  [unwired: 2 in, 2 out]
        n283 = call "IMAQ ColorThreshold"("Blue or Luma or Val or Inten Range"=w500, "Replace Value"=w486, "Green or Sat Range"=w499, "Color Mode"=w497, "Red or Hue Range"=w498, "Image Dst"=w496, "Image Src"=w444) -> ("Image Dst Out"=w485:T1)  [unwired: 3 in, 1 out]
        n284 = call-poly <vilib>:"SD Write Value.vi"("Numeric"="Tiempo de Espera", "Name"="time to wait") -> ()  [unwired: 8 in, 2 out]
        n285 = call "IMAQ ColorThreshold"("Blue or Luma or Val or Inten Range"=w467, "Replace Value"=w458, "Green or Sat Range"=w466, "Color Mode"=w464, "Red or Hue Range"=w465, "Image Dst"=w450, "Image Src"=w443) -> ("Image Dst Out"=w457:T1)  [unwired: 3 in, 1 out]
        n286 = Bundle("Color Box"=w506, "Color Box"=w506) -> (w508:cluster{"Color Box":u32, "Color Box":u32})  [unwired: 1 out]
        n287 = call "Sorted Particle Report 2015.vi"("Min Area Size %"=w492, "Particle Count Limit"=w495, "Pixel Measurements"=w451, "Image in"=w485) -> ("Sorted Data"=w493:dbl[][], "Particles"=→"Particles":i32)
        n288 = Build Array(w508) -> (w507:cluster{"Color Box":u32, "Color Box":u32}[])
        n289 = property on="Mbps 2" class="Bool (strict)"("Colors [4]"=w507) -> ()  [unwired: 2 in, 2 out]
        n290 = call "Sorted Particle Report 2015.vi"("Min Area Size %"=w460, "Particle Count Limit"=w463, "Pixel Measurements"=w451, "Image in"=w457) -> ("Sorted Data"=w461:dbl[][], "Particles"=→"Particles 2":i32)
        n291 = call "Calculate Particle Scores.vi"("Pixel Value"=w486, "Limit Tests?"="Limit Tests?", "Aspect Fudge Factor"="Aspect Fudge Factor", "Sorted Data"=w493, "Image in"=w485) -> ("Scores"=w488:T32)  [unwired: 6 in]
        n292 = call "Calculate Particle Scores.vi"("Pixel Value"=w458, "Limit Tests?"="Limit Tests?", "Aspect Fudge Factor"="Aspect Fudge Factor", "Sorted Data"=w461, "Image in"=w457) -> ("Scores"=w459:T32)  [unwired: 6 in]
        n293 = flat-sequence {
          tunnel: w488 -> [w512]
          tunnel: [w512] -> w487
          frame #0 {
            # "Evaluate and rank based\non goals and strategy?"
          }
        }
        n294 = flat-sequence {
          tunnel: w459 -> [w511]
          tunnel: [w511] -> w453
          frame #0 {
            # "Evaluate and rank based\non goals and strategy?"
          }
        }
        n295 = Bundle("Red"="Red", "Blue"="Blue") -> (w470:T33)  [unwired: 1 in]
        n296 = call "Check for Carpet.vi"("Original Mask"=w485, "Original Color"=w444, "Carpet Colors"=w470, "Carpet Selector"="Carpet Color", "Combine Carpet Mask"="Show Carpet Mask", "Initial Scores"=w487) -> ("Updated Mask"=→"Masked":T1, "Updated Scores"=w484:T34)  [unwired: 4 in]
        n297 = call "Check for Carpet.vi"("Original Mask"=w457, "Original Color"=w443, "Carpet Colors"=w470, "Carpet Selector"="Carpet Color", "Combine Carpet Mask"="Show Carpet Mask", "Initial Scores"=w453) -> ("Updated Mask"=→"Extracted Masked":T1, "Updated Scores"=w456:T34)  [unwired: 4 in]
        n298 = call "Label Targets2.vi"("Score Threshold"="Score Threshold", "Annotate"="Annotate", "Targets"=w456, "Image in"=w443) -> ("Image out"=→"Original Extracted":T1)  [unwired: 7 in]
        n299 = call "Normalize Coordinates.vi"("Camera Type"="Camera Type", "Targets"=w456, "Image in"=w443) -> ("Found Totes"=w437:T8, "Sorted Scores"=→"Sorted Scores Extracted":T9)  [unwired: 7 in]
        "Detected Totes Extracted" <- w437
        "Found Totes" <- w437
        n300 = call "Label Targets2.vi"("Score Threshold"="Score Threshold", "Annotate"="Annotate", "Targets"=w484, "Image in"=w444) -> ("Image out"=→"Original Image":T1)  [unwired: 7 in]
        n301 = call "Normalize Coordinates.vi"("Camera Type"="Camera Type", "Targets"=w484, "Image in"=w444) -> ("Found Totes"=w481:T8, "Sorted Scores"=→"Sorted Scores":T9)  [unwired: 7 in]
        "Detected Totes" <- w481
        n302 = Array To Cluster(array=w437) -> (cluster=w436:T35)
        n303 = Array To Cluster(array=w481) -> (cluster=w482:T35)
        n304 = Unbundle By Name(w436) -> ("Found Totes[0].Normalized Rect.Numeric"=w435:dbl, "Found Totes[0].Normalized Rect.Numeric 2"=w434:dbl, "Found Totes[0].Normalized Rect.Numeric 3"=w433:dbl, "Found Totes[0].Normalized Rect.Numeric 5"=w432:dbl)
        n305 = Unbundle By Name(w482) -> ("Found Totes[0].Center"=w479:cluster{dbl, dbl})
        n306 = Unbundle(w479) -> (w478:dbl)  [unwired: 1 out]
        n307 = Not Equal To 0?(x=w435) -> (x != 0?=w431:bool)
        n308 = Not Equal To 0?(x=w434) -> (x != 0?=w430:bool)
        n309 = Not Equal To 0?(x=w433) -> (x != 0?=w429:bool)
        n310 = Not Equal To 0?(x=w432) -> (x != 0?=w428:bool)
        n311 = Compound Arithmetic op=OR(w431, w430, w429, w428) -> (w426:bool)
        n312 = call-poly <vilib>:"SD Write Value.vi"("Boolean"=w426, "Name"="puedo recoger") -> ()  [unwired: 8 in, 2 out]
        n313 = call-poly <vilib>:"SD Write Value.vi"("Numeric"=w478, "Name"="center") -> ()  [unwired: 8 in, 2 out]
        "Mbps" <- w505
        "fps" <- w504
      }
    }
  }
  n314 = while {
    tunnel: w17 -> [w517]
    stop <- FALSE stop-if-true
    n315 = TCP Wait On Listener(11:w517) -> (4:w516:refnum<k5>)  [unwired: 3 in, 4 out]
    n316 = local write "TCP"(w516) -> ()
  }
  n317 = property on="On/Off" class="Bool (strict)"("Visible"=w22) -> ()  [unwired: 2 in, 2 out]
  n318 = property on="Motor" class="Clust (strict)"("Visible"=w22) -> ()  [unwired: 2 in, 2 out]
  n319 = property on="Progress" class="Clust (strict)"("Visible"=w22) -> ()  [unwired: 2 in, 2 out]
  n320 = property on="Test Ring" class="Ring (strict)"("Visible"=w22) -> ()  [unwired: 2 in, 2 out]
  n321 = property on="Rev/Fwd" class="Clust (strict)"("Visible"=w22) -> ()  [unwired: 2 in, 2 out]
  n322 = property on="Camera Settings" class="Clust (strict)"("Visible"=w22) -> ()  [unwired: 2 in, 2 out]
  n323 = local write "DB Camera Config"(w22) -> ()
  n324 = global write "WPI_DashboardLogging Global.vi" "Recording"(w46) -> ()
  n325 = local write "Rec Mode"(w46) -> ()
